vi "Setup Multi Acq No Objects.vi"(6 "# of Scans":u32, 7 "Time Between Acq (ms)":u32, 8 "Cosmic Ray Removal?":bool=TRUE, 9 "Averaging?":bool, 10 "Dark Subtract?":bool, 11 "Synapse CCD in":T1={"JYCCDLib.IJYCCDReqd"=refnum, "JYMONOLib.IJYMonoReqd"=refnum, "Integration time"=0.01, "ADC"=0, "GAIN"=0, "areas :"=[[1, 1, 1, 1024, 256, 1, 256]], "Most Recent Data Object"=refnum, "Mono Properties"={"Grating"=0, "Center Wavelength"=0.0, "Entrance Slit"=0.0, "Exit Slit"=0.0}, "Coverage"={"Max"=0.0, "Min"=0.0}, "Multi-Acquisitions"={"Dark Subtract?"=FALSE, "Averaging?"=FALSE, "Cosmic Ray Removal?"=FALSE, "# to Average"=0, "Time Between Acq."=0, "Acquisitions Control Array"=[TRUE], "Raw Data"=[], "Processed Data"=[], "Array of Wavelengths"=[]}, "Channel Names"=["Wavelength", "Signal"], "Channel Units"=["nm", "counts"]} {"ADC" items=["   20 kHz", "1 MHz", "1 MHz Ultra"]; "GAIN" items=["High Light", "Best Dynamic", "High Sensitivity"]; "Mono Properties"."Grating" items=["1200 lines/mm - 500 nm Blaze", "1200 lines/mm - 750 nm Blaze", "600 lines/mm - 1000 nm Blaze"]}) -> (3 "Synapse CCD out":T1={"JYCCDLib.IJYCCDReqd"=refnum, "JYMONOLib.IJYMonoReqd"=refnum, "Integration time"=0.01, "ADC"=0, "GAIN"=0, "areas :"=[[1, 1, 1, 1024, 256, 1, 256]], "Most Recent Data Object"=refnum, "Mono Properties"={"Grating"=0, "Center Wavelength"=0.0, "Entrance Slit"=0.0, "Exit Slit"=0.0}, "Coverage"={"Max"=0.0, "Min"=0.0}, "Multi-Acquisitions"={"Dark Subtract?"=FALSE, "Averaging?"=FALSE, "Cosmic Ray Removal?"=FALSE, "# to Average"=0, "Time Between Acq."=0, "Acquisitions Control Array"=[TRUE], "Raw Data"=[], "Processed Data"=[], "Array of Wavelengths"=[]}, "Channel Names"=["Wavelength", "Signal"], "Channel Units"=["nm", "counts"]} {"ADC" items=["   20 kHz", "1 MHz", "1 MHz Ultra"]; "GAIN" items=["High Light", "Best Dynamic", "High Sensitivity"]; "Mono Properties"."Grating" items=["1200 lines/mm - 500 nm Blaze", "1200 lines/mm - 750 nm Blaze", "600 lines/mm - 1000 nm Blaze"]})   [LabVIEW 2012]
doc: "Loads Multi-Acq parameters into member data and creates Boolean Control Array for member data."
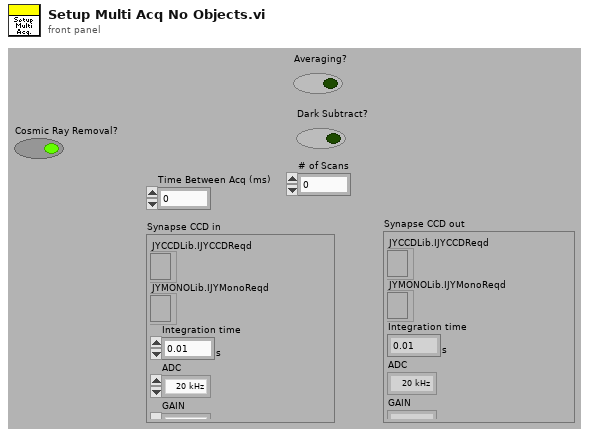
[diagram p1: front panel]
types:
  T1 = cluster{"JYCCDLib.IJYCCDReqd":refnum<k7>, "JYMONOLib.IJYMonoReqd":refnum<k7>, "Integration time":dbl[unit], "ADC":u16, "GAIN":u16, "areas :":i32[][], "Most Recent Data Object":refnum<k7>, "Mono Properties":cluster{"Grating":u16, "Center Wavelength":dbl[unit], "Entrance Slit":dbl[unit], "Exit Slit":dbl[unit]}, "Coverage":cluster{"Max":dbl[unit], "Min":dbl[unit]}, "Multi-Acquisitions":cluster{"Dark Subtract?":bool, "Averaging?":bool, "Cosmic Ray Removal?":bool, "# to Average":u32, "Time Between Acq.":u32, "Acquisitions Control Array":bool[], "Raw Data":i32[][], "Processed Data":dbl[], "Array of Wavelengths":dbl[]}, "Channel Names":string[], "Channel Units":string[]}
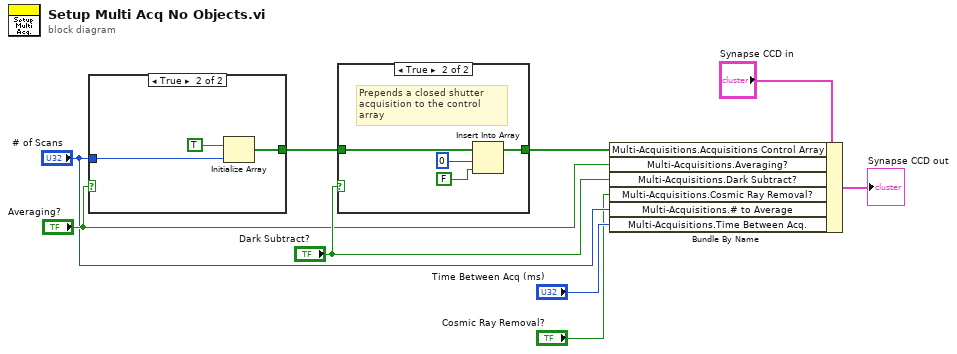
[diagram p0: block diagram]
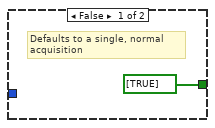
[diagram p3: hidden frame]
diagram:
  n1 = case shown="True" "Averaging?" {
    tunnel: [bool[] [TRUE] w12] -> w9
    tunnel: "# of Scans" -> [_ w11]
    frame False {
      # "Defaults to a single, normal\nacquisition"
    }
    frame True {
      n2 = Initialize Array(TRUE, w11) -> (w12:bool[])
    }
  }
  n3 = case shown="True" "Dark Subtract?" {
    tunnel: w9 -> [w14 w18]
    tunnel: [w14 w15] -> w8
    frame False {
    }
    frame True {
      # "Prepends a closed shutter\nacquisition to the control\narray"
      n4 = Insert Into Array(array=w18, index=0, new element=FALSE) -> (w15:bool[])
    }
  }
  n5 = Bundle By Name(cluster="Synapse CCD in", "Multi-Acquisitions.Acquisitions Control Array"=w8, "Multi-Acquisitions.Averaging?"="Averaging?", "Multi-Acquisitions.Dark Subtract?"="Dark Subtract?", "Multi-Acquisitions.Cosmic Ray Removal?"="Cosmic Ray Removal?", "Multi-Acquisitions.# to Average"="# of Scans", "Multi-Acquisitions.Time Between Acq."="Time Between Acq (ms)") -> (→"Synapse CCD out":T1)
